vi "Lecture All clef of section Software.vi"(8 "error in (no error)":errorcluster caption="entrée d'erreur (pas d'erreur)", 10 "File et Queue":T2) -> (0 "error out":errorcluster caption="sortie d'erreur", 1 "Multi Produit":bool, 2 "Display":cluster{"CheckBox PCB":T1, "CheckBox PCBA":T1}, 3 "Commande chemin":path)   [LabVIEW 2020]
uses:
  File et notificateur/File et notification.ctl
  TypeDef/Data Event Sequenceur.ctl
  TypeDef/Liste Event Sequenceur.ctl
  TypeDef/Liste Fonction appelante.ctl
  Tache Generation Historique/Type DEF/Data Event Historique.ctl
  Tache Generation Historique/Type DEF/Liste Event Historique.ctl
  Type DEF/Commande Selection produit en cours.ctl
  TypeDef/Commande Variable Global.ctl
  Type DEF/Commande Variables Programme.ctl
  Type DEF/Commande tableau Resultat.ctl
  Instrument/BLE/Comande Variable Globale BLE.ctl
  Drivers/BLE/type_def/connection_status_bundle.ctl
  Drivers/BLE/type_def/address_type.ctl
  Type DEF/Commande Event Demande Op.ctl
  Type DEF/Commande Event Demande Autotest.ctl
  Type DEF/Commande Action Lecture RS Bridge.ctl
  Type DEF/Commande Event Saisie Op.ctl
  TypeDef/Liste fonction Saisie Operateur.ctl
  Type DEF/Commande Event Affiche Result.ctl
  Fonction/Shielding Box/Action.ctl
  TypeDef/Adresse IHM.ctl
  Commande special/CheckBox 2.ctl
  <vilib>/Utility/config.llb/Read Key (String).vi
  <vilib>/Utility/config.llb/Read Key (Path).vi
  <vilib>/Utility/config.llb/Read Key (U32).vi
  <vilib>/Utility/config.llb/NI_LVConfig.lvlib
  Commun VI/Library Commun.lvlib
panel:
  # "Application"
  # "Sequenceur"
  # "Data"
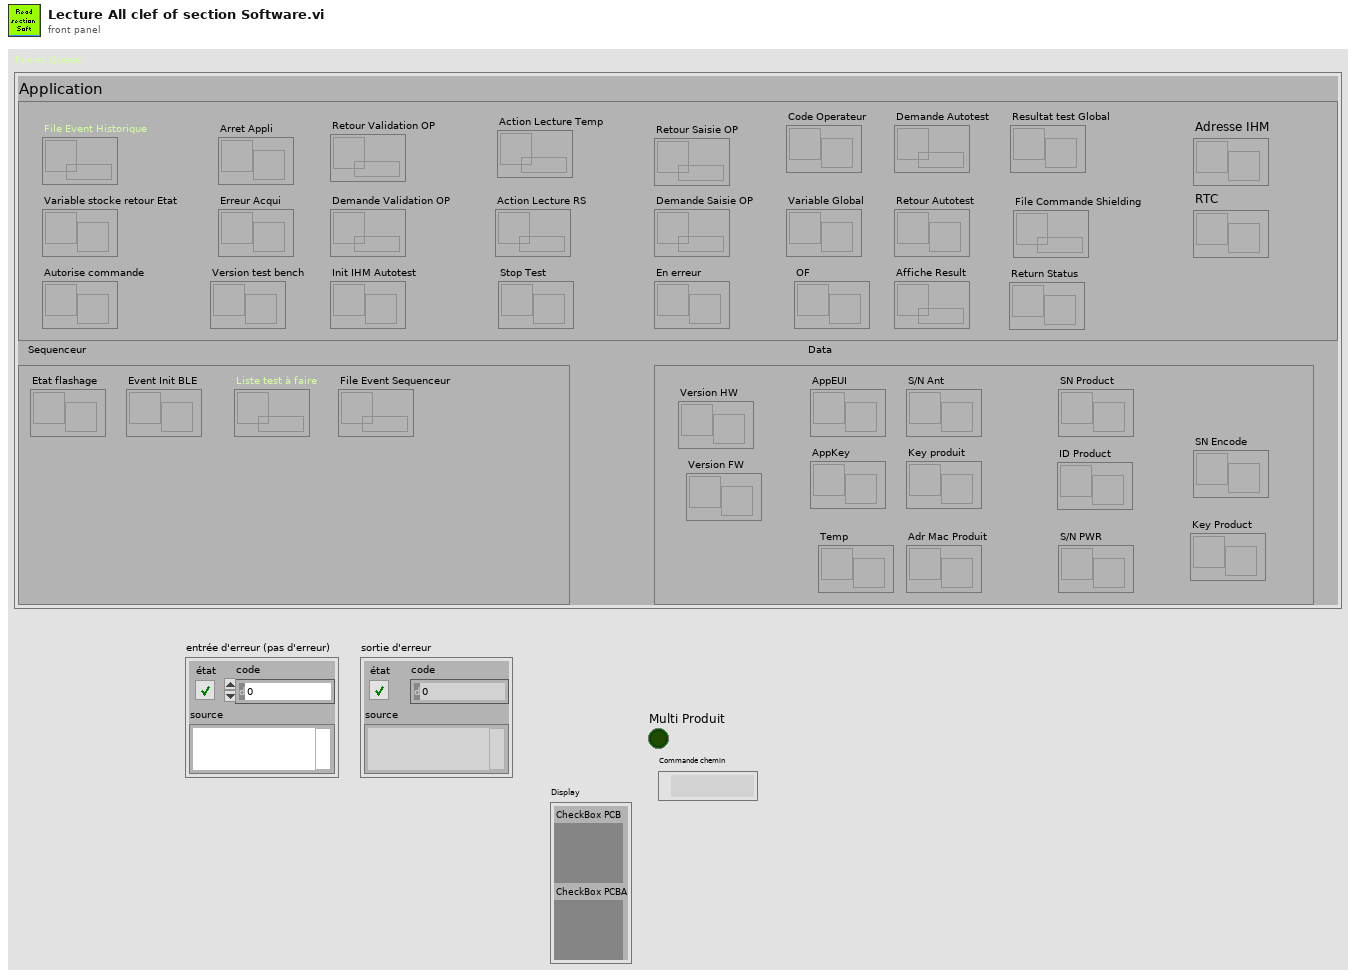
[diagram p1: front panel]
types:
  T1 = typedef "CheckBox 2.ctl" = u16
  T2 = typedef "File et notification.ctl" = cluster{"Arret Appli":refnum<notifier>, "Erreur Acqui":refnum<notifier>, "File Event Sequenceur":refnum<queue>, "Liste test à faire":refnum<queue>, "File Event Historique":refnum<queue>, "Variable Global":refnum<notifier>, "Variable stocke retour Etat":refnum<notifier>, "Retour Validation OP":refnum<queue>, "Demande Validation OP":refnum<queue>, "Retour Autotest":refnum<notifier>, "Demande Autotest":refnum<queue>, "Adr Mac Produit":refnum<notifier>, "Autorise commande":refnum<notifier>, "Event Init BLE":refnum<notifier>, "Action Lecture RS":refnum<queue>, "Key produit":refnum<notifier>, "Retour Saisie OP":refnum<queue>, "Demande Saisie OP":refnum<queue>, "Etat flashage":refnum<notifier>, "Code Operateur":refnum<notifier>, "Resultat test Global":refnum<notifier>, "Stop Test":refnum<notifier>, "Init IHM Autotest":refnum<notifier>, "Version test bench":refnum<notifier>, "SN Product":refnum<notifier>, "En erreur":refnum<notifier>, "Affiche Result":refnum<queue>, "S/N PWR":refnum<notifier>, "AppEUI":refnum<notifier>, "Action Lecture Temp":refnum<queue>, "Temp":refnum<notifier>, "AppKey":refnum<notifier>, "OF":refnum<notifier>, "File Commande Shielding":refnum<queue>, "Return Status":refnum<notifier>, "ID Product":refnum<notifier>, "Version FW":refnum<notifier>, "Version HW":refnum<notifier>, "Adresse IHM":refnum<notifier>, "RTC":refnum<notifier>, "S/N Ant":refnum<notifier>, "SN Encode":refnum<notifier>, "Key Product":refnum<notifier>}
  T3 = cluster{"Date":string, "Version":string, "Titre":string, "Fichier Application":string}
  T4 = typedef "NI_LVConfig.lvlib/Config Data RefNum.ctl" = refnum<k1>
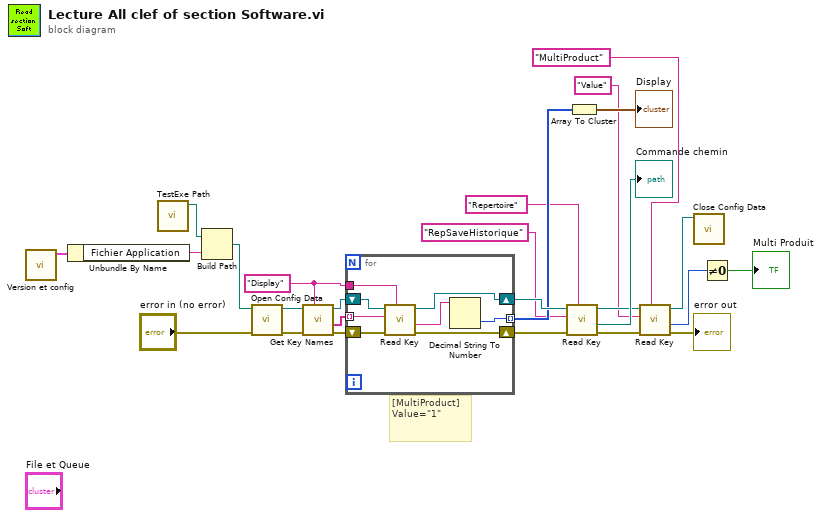
[diagram p0: block diagram]
diagram:
  w16 = "Display" ("nom ou chemin relatif")
  # "[MultiProduct]\nValue=\"1\""
  n1 = call "Version et config.vi"() -> ("OutPut"=w3:T3)  [unwired: 11 in]
  n2 = Unbundle By Name(w3) -> ("Fichier Application"=w2:string)
  n3 = call "TestExe Path.vi"() -> ("Chemin Actuel"=w1:path)  [unwired: 9 in, 2 out]
  n4 = Build Path(base path=w1, name or relative path=w2) -> (appended path=w26:path)
  n5 = call <vilib>:"Open Config Data.vi"("error in (no error)"="error in (no error)", "configuration file path"=w26) -> ("error out"=w25:errorcluster, "refnum"=w23:T4)  [unwired: 7 in, 1 out]
  n6 = call <vilib>:"Get Key Names.vi"("section"=w16, "error in (no error)"=w25, "refnum"=w23) -> ("error out"=w24:errorcluster, "key names"=w21:string[], "refnum out"=w22:T4)  [unwired: 5 in, 1 out]
  n7 = for {
    shift-right: [w31] -> w19
    shift-left: w22 -> [w34]
    shift-right: [w32] -> w20
    shift-left: w24 -> [w33]
    tunnel: [w27] -> w18 mode=indexing
    tunnel: w21 -> [w29] mode=indexing
    tunnel: w16 -> [w28]
    n8 = call-poly <vilib>:"Read Key.vi"("section"=w28, "error in (no error)"=w33, "key"=w29, "refnum"=w34) -> ("error out"=w32:errorcluster, "value"=w30:string, "refnum out"=w31:T4)  [unwired: 4 in, 1 out]
    n9 = Decimal String To Number(string=w30) -> (number=w27:i32)  [unwired: 2 in, 1 out]
  }
  n10 = call-poly <vilib>:"Read Key.vi"("section"="Repertoire" ("nom ou chemin relatif"), "error in (no error)"=w20, "key"="RepSaveHistorique", "refnum"=w19) -> ("error out"=w10:errorcluster, "value"=→"Commande chemin":path, "refnum out"=w12:T4)  [unwired: 4 in, 1 out]
  n11 = Array To Cluster(array=w18) -> (cluster=→"Display":cluster{"[0]":i32, "[1]":i32})
  n12 = call-poly <vilib>:"Read Key.vi"("section"="MultiProduct" ("nom ou chemin relatif"), "error in (no error)"=w10, "key"="Value", "refnum"=w12) -> ("error out"=→"error out":errorcluster, "value"=w6:u32, "refnum out"=w11:T4)  [unwired: 4 in, 1 out]
  n13 = call <vilib>:"Close Config Data.vi"("refnum"=w11) -> ()  [unwired: 9 in, 2 out]
  n14 = Not Equal To 0?(x=w6) -> (x != 0?=→"Multi Produit":bool)
